vi "sv_Integrate and Differentiate Units.vi"(5 "integration type":T1(ring)=enum."none", 7 "custom unit label in":string, 8 "engineering units in":T2 items=["custom..."=0, "V"=1, "A"=21, "C"=30, "pC"=31, "s"=32, "-"=29, "Pa"=2, "N"=20, "g"=3, "m/s^2"=4, "m/s"=5, "m"=6, "mm/s"=12, "mm"=13, "micron/s"=14, "micron"=15, "in/s^2"=7, "in/s"=8, "in"=9, "mil/s"=10, "mil"=11, "rad/s^2"=16, "rad/s"=17, "rad"=18, "deg/s^2"=26, "deg/s"=27, "deg"=28, "RPM"=22, "cycle/s^2"=23, "Hz"=24, "cycle"=25, "strain"=19], 9 "input value":dbl=1.0) -> (1 "custom unit label out":string, 2 "engineering units out":T2 items=["custom..."=0, "V"=1, "A"=21, "C"=30, "pC"=31, "s"=32, "-"=29, "Pa"=2, "N"=20, "g"=3, "m/s^2"=4, "m/s"=5, "m"=6, "mm/s"=12, "mm"=13, "micron/s"=14, "micron"=15, "in/s^2"=7, "in/s"=8, "in"=9, "mil/s"=10, "mil"=11, "rad/s^2"=16, "rad/s"=17, "rad"=18, "deg/s^2"=26, "deg/s"=27, "deg"=28, "RPM"=22, "cycle/s^2"=23, "Hz"=24, "cycle"=25, "strain"=19], 3 "output value":dbl)   [LabVIEW 2017]
uses:
  <vilib>/addons/_NISVFA/_Shared subVIs/Controls/svc_Engineering Units Text Ring.ctl
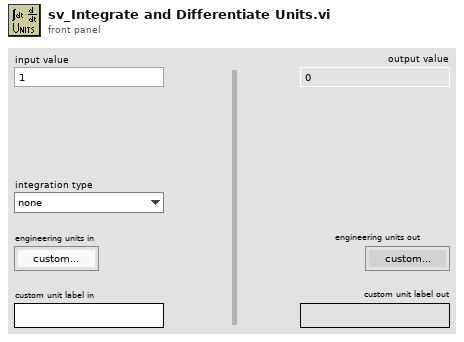
[diagram p1: front panel]
types:
  T1 = enum16{"single integration", "double integration", "single differentiation", "double differentiation", "none"}
  T2 = typedef "svc_Engineering Units Text Ring.ctl" = u16
  T3 = enum16{"custom...", "V", "Pa", "g", "m/s^2", "m/s", "m", "in/s^2", "in/s", "in", "mil/s", "mil", "mm/s", "mm", "micron/s", "micron", "rad/s^2", "rad/s", "rad", "strain", "N", "A", "rpm", "cycle/s^2", "Hz", "cycle", "deg/s^2", "deg/s", "deg", "Undefined", "C", "pC"}
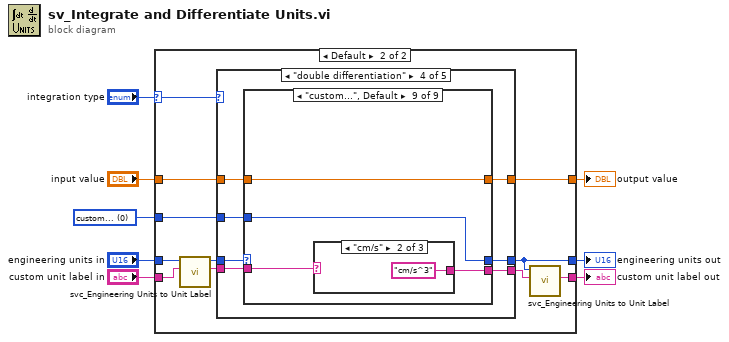
[diagram p0: block diagram]
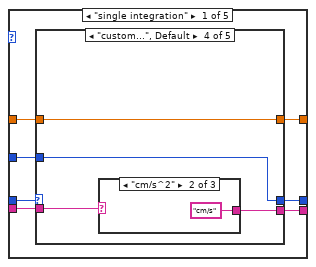
[diagram p3: hidden frame]
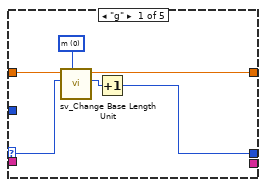
[diagram p4: hidden frame]
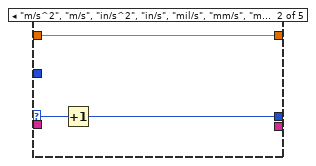
[diagram p5: hidden frame]
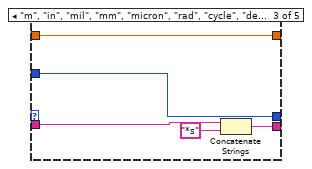
[diagram p6: hidden frame]
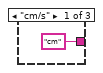
[diagram p7: hidden frame]
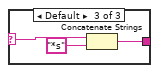
[diagram p8: hidden frame]
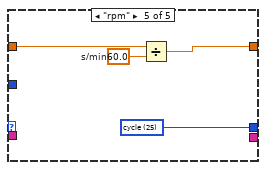
[diagram p9: hidden frame]
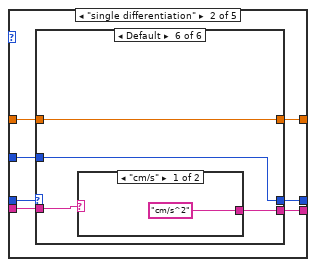
[diagram p10: hidden frame]
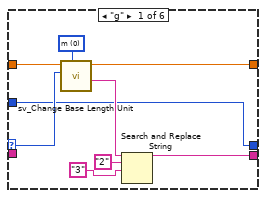
[diagram p11: hidden frame]
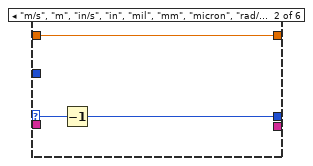
[diagram p12: hidden frame]
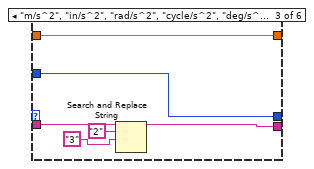
[diagram p13: hidden frame]
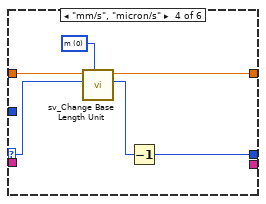
[diagram p14: hidden frame]
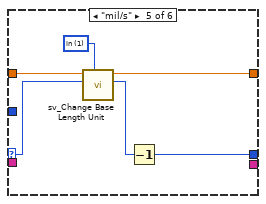
[diagram p15: hidden frame]
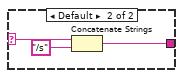
[diagram p16: hidden frame]
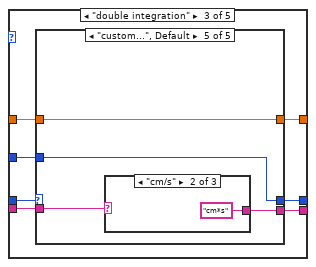
[diagram p17: hidden frame]
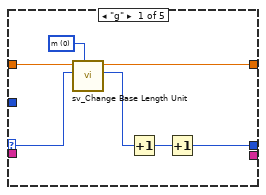
[diagram p18: hidden frame]
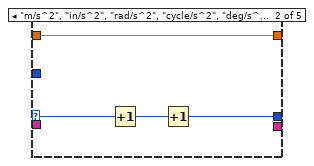
[diagram p19: hidden frame]
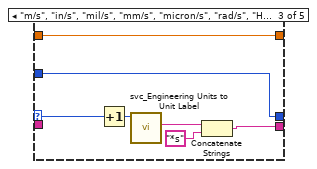
[diagram p20: hidden frame]
diagram:
  w1 = T2 0 items=["custom..."=0, "V"=1, "A"=21, "Pa"=2, "N"=20, "g"=3, "m/s^2"=4, "m/s"=5, "m"=6, "mm/s"=12, "mm"=13, "micron/s"=14, "micron"=15, "in/s^2"=7, "in/s"=8, "in"=9, "mil/s"=10, "mil"=11, "rad/s^2"=16, "rad/s"=17, "rad"=18, "deg/s^2"=26, "deg/s"=27, "deg"=28, "RPM"=22, "cycle/s^2"=23, "Hz"=24, "cycle"=25, "strain"=19] ("engineering units")
  n1 = case shown="Default" "integration type" {
    selector: "integration type" -> [_ w14]
    tunnel: [w9 w22] -> w8
    tunnel: [w10 w20] -> w7
    tunnel: "custom unit label in" -> [w9 w18]
    tunnel: [w11 w17] -> w5
    tunnel: "input value" -> [w11 w16]
    tunnel: "engineering units in" -> [w10 w13]
    tunnel: w1 -> [_ w12]
    frame "none" {
    }
    frame Default {
      n2 = call <vilib>:"svc_Engineering Units to Unit Label.vi"("custom label"=w18, "engineering units"=w13) -> ("unit label"=w19:string, "engineering units enum"=w15:T3)  [unwired: 8 in]
      n3 = case shown="\"double differentiation\"" w14 {
        tunnel: w15 -> [w29 w57 w108 w147 _]
        tunnel: [w28 w63 w107 w146 w221] -> w17
        tunnel: w16 -> [w27 w62 w106 w145 w221]
        tunnel: w19 -> [w26 w61 w105 w144 w220]
        tunnel: [w25 w60 w104 w143 _] -> w20
        tunnel: [w23 w58 w103 w142 w220] -> w21
        tunnel: w12 -> [w24 w59 w102 w141 _]
        frame "single integration" {
          n4 = case shown="\"custom...\", Default" w29 {
            selector: w29 -> [w32 w38 _ _ _]
            tunnel: [w34 w37 w39 w45 w53] -> w28
            tunnel: w27 -> [w35 w37 w39 w45 w54]
            tunnel: w26 -> [_ _ w40 w44 _]
            tunnel: [w33 w36 w42 w47 w56] -> w25
            tunnel: w24 -> [_ _ w42 w47 _]
            tunnel: [_ _ w41 w46 _] -> w23
            frame "g" {
              w31 = 0 items=["no change"=-1, "m"=0, "mm"=2, "microns"=3, "in"=1, "mils"=5] ("desired base units for length")
              n5 = call <vilib>:"sv_Change Base Length Unit.vi"("desired base units for vibration"=w31, "engineering units in"=w32, "value in [EU]"=w35) -> ("engineering units out"=w30:T2, "value out [desired EU]"=w34:dbl)  [unwired: 4 in, 1 out]
              n6 = Increment(x=w30) -> (x+1=w33:T2)
            }
            frame "m/s^2", "m/s", "in/s^2", "in/s", "mil/s", "mm/s", "micron/s", "rad/s^2", "rad/s", "cycle/s^2", "Hz", "deg/s^2", "deg/s" {
              n7 = Increment(x=w38) -> (x+1=w36:T3)
            }
            frame "m", "in", "mil", "mm", "micron", "rad", "cycle", "deg" {
              n8 = Concatenate Strings(w40, "*s" ("Input Element")) -> (w41:string)
            }
            frame "custom...", Default {
              n9 = case shown="\"cm/s^2\"" w44 {
                selector: w44 -> [_ _ w50]
                tunnel: ["cm" "cm/s" w51] -> w46
                frame "cm/s" {
                }
                frame "cm/s^2" {
                }
                frame Default {
                  n10 = Concatenate Strings(w50, "*s" ("Input Element")) -> (w51:string)
                }
              }
            }
            frame "rpm" {
              w55 = 60.0  # s/min
              w56 = T2 25 items=["custom..."=0, "V"=1, "A"=21, "Pa"=2, "N"=20, "g"=3, "m/s^2"=4, "m/s"=5, "m"=6, "mm/s"=12, "mm"=13, "micron/s"=14, "micron"=15, "in/s^2"=7, "in/s"=8, "in"=9, "mil/s"=10, "mil"=11, "rad/s^2"=16, "rad/s"=17, "rad"=18, "deg/s^2"=26, "deg/s"=27, "deg"=28, "RPM"=22, "cycle/s^2"=23, "Hz"=24, "cycle"=25, "strain"=19] ("engineering units")
              n11 = Divide(x=w54, y=w55) -> (x/y=w53:dbl)
            }
          }
        }
        frame "single differentiation" {
          n12 = case shown="Default" w57 {
            selector: w57 -> [w69 w75 _ w84 w90 _]
            tunnel: [w71 w74 w80 w86 w92 w95] -> w63
            tunnel: w62 -> [w72 w74 w80 w87 w93 w95]
            tunnel: w61 -> [_ _ w79 _ _ w94]
            tunnel: [w64 w73 w81 w82 w88 w97] -> w60
            tunnel: w59 -> [w64 _ w81 _ _ w97]
            tunnel: [w70 _ w78 _ _ w96] -> w58
            frame "g" {
              w68 = 0 items=["no change"=-1, "m"=0, "mm"=2, "microns"=3, "in"=1, "mils"=5] ("desired base units for length")
              n13 = call <vilib>:"sv_Change Base Length Unit.vi"("desired base units for vibration"=w68, "engineering units in"=w69, "value in [EU]"=w72) -> ("custom label out"=w65:string, "value out [desired EU]"=w71:dbl)  [unwired: 4 in, 1 out]
              n14 = Search and Replace String(input string=w65, search string="2", replace string="3" ("replace string (\"\")")) -> (result string=w70:string)  [unwired: 5 in, 3 out]
            }
            frame "m/s", "m", "in/s", "in", "mil", "mm", "micron", "rad/s", "rad", "Hz", "cycle", "deg/s", "deg" {
              n15 = Decrement(x=w75) -> (x-1=w73:T3)
            }
            frame "m/s^2", "in/s^2", "rad/s^2", "cycle/s^2", "deg/s^2" {
              n16 = Search and Replace String(input string=w79, search string="2", replace string="3" ("replace string (\"\")")) -> (result string=w78:string)  [unwired: 5 in, 3 out]
            }
            frame "mm/s", "micron/s" {
              w85 = 0 items=["no change"=-1, "g"=386, "m"=0, "cm"=4, "mm"=2, "microns"=3, "in"=1, "mils"=5] ("desired base units for vibration")
              n17 = call <vilib>:"sv_Change Base Length Unit.vi"("desired base units for vibration"=w85, "engineering units in"=w84, "value in [EU]"=w87) -> ("engineering units out"=w83:T2, "value out [desired EU]"=w86:dbl)  [unwired: 4 in, 1 out]
              n18 = Decrement(x=w83) -> (x-1=w82:T2)
            }
            frame "mil/s" {
              w91 = 1 items=["no change"=-1, "g"=386, "m"=0, "cm"=4, "mm"=2, "microns"=3, "in"=1, "mils"=5] ("desired base units for vibration")
              n19 = call <vilib>:"sv_Change Base Length Unit.vi"("desired base units for vibration"=w91, "engineering units in"=w90, "value in [EU]"=w93) -> ("engineering units out"=w89:T2, "value out [desired EU]"=w92:dbl)  [unwired: 4 in, 1 out]
              n20 = Decrement(x=w89) -> (x-1=w88:T2)
            }
            frame Default {
              n21 = case shown="\"cm/s\"" w94 {
                selector: w94 -> [_ w99]
                tunnel: ["cm/s^2" w100] -> w96
                frame "cm/s" {
                }
                frame Default {
                  n22 = Concatenate Strings(w99, "/s" ("Input Element")) -> (w100:string)
                }
              }
            }
          }
        }
        frame "double integration" {
          n23 = case shown="\"custom...\", Default" w108 {
            selector: w108 -> [w113 w118 w126 _ _]
            tunnel: [w115 w119 w125 w131 w135] -> w107
            tunnel: w106 -> [w114 w119 w125 w131 w135]
            tunnel: w105 -> [_ _ _ w127 w132]
            tunnel: [w109 w116 w124 w130 w134] -> w104
            tunnel: [_ _ w120 w129 w133] -> w103
            tunnel: w102 -> [_ _ w124 w130 w134]
            frame "g" {
              w112 = 0 items=["no change"=-1, "m"=0, "mm"=2, "microns"=3, "in"=1, "mils"=5] ("desired base units for length")
              n24 = call <vilib>:"sv_Change Base Length Unit.vi"("desired base units for vibration"=w112, "engineering units in"=w113, "value in [EU]"=w114) -> ("engineering units out"=w111:T2, "value out [desired EU]"=w115:dbl)  [unwired: 4 in, 1 out]
              n25 = Increment(x=w111) -> (x+1=w110:T2)
              n26 = Increment(x=w110) -> (x+1=w109:T2)
            }
            frame "m/s^2", "in/s^2", "rad/s^2", "cycle/s^2", "deg/s^2" {
              n27 = Increment(x=w118) -> (x+1=w117:T3)
              n28 = Increment(x=w117) -> (x+1=w116:T3)
            }
            frame "m/s", "in/s", "mil/s", "mm/s", "micron/s", "rad/s", "Hz", "deg/s" {
              n29 = Increment(x=w126) -> (x+1=w121:T3)
              n30 = call <vilib>:"svc_Engineering Units to Unit Label.vi"("engineering units"=w121) -> ("unit label"=w122:string)  [unwired: 9 in, 1 out]
              n31 = Concatenate Strings(w122, "*s" ("custom label")) -> (w120:string)
            }
            frame "m", "in", "mil", "mm", "micron", "rad", "cycle", "deg" {
              n32 = Concatenate Strings(w127, "*s^2" ("custom label")) -> (w129:string)
            }
            frame "custom...", Default {
              n33 = case shown="\"cm/s\"" w132 {
                selector: w132 -> [_ _ w138]
                tunnel: ["cm" "cm*s" w140] -> w133
                frame "cm/s^2" {
                }
                frame "cm/s" {
                }
                frame Default {
                  n34 = Concatenate Strings(w138, "*s^2" ("custom label")) -> (w140:string)
                }
              }
            }
          }
        }
        frame "double differentiation" {
          n35 = case shown="\"custom...\", Default" w147 {
            selector: w147 -> [w153 _ w170 w172 w183 w195 w199 w206 _]
            tunnel: [w156 w162 w169 w173 w184 w196 w200 w207 w212] -> w146
            tunnel: w145 -> [w155 w162 w169 w174 w185 w196 w201 w208 w212]
            tunnel: w144 -> [_ w158 _ _ _ _ _ _ w211]
            tunnel: [w154 w161 w168 w181 w192 w193 w202 w209 w213] -> w143
            tunnel: [w148 w157 w163 w176 w187 _ _ _ w214] -> w142
            tunnel: w141 -> [w154 w161 w168 w181 w192 _ _ _ w213]
            frame "g" {
              w152 = 0 items=["no change"=-1, "m"=0, "mm"=2, "microns"=3, "in"=1, "mils"=5] ("desired base units for length")
              n36 = call <vilib>:"sv_Change Base Length Unit.vi"("desired base units for vibration"=w152, "engineering units in"=w153, "value in [EU]"=w155) -> ("custom label out"=w149:string, "value out [desired EU]"=w156:dbl)  [unwired: 4 in, 1 out]
              n37 = Search and Replace String(input string=w149, search string="2", replace string="4" ("replace string (\"\")")) -> (result string=w148:string)  [unwired: 5 in, 3 out]
            }
            frame "m/s^2", "in/s^2", "rad/s^2", "cycle/s^2", "deg/s^2" {
              n38 = Search and Replace String(input string=w158, search string="2", replace string="4" ("replace string (\"\")")) -> (result string=w157:string)  [unwired: 5 in, 3 out]
            }
            frame "m/s", "in/s", "rad/s", "Hz", "deg/s" {
              n39 = Decrement(x=w170) -> (x-1=w167:T3)
              n40 = call <vilib>:"svc_Engineering Units to Unit Label.vi"("engineering units"=w167) -> ("unit label"=w164:string)  [unwired: 9 in, 1 out]
              n41 = Search and Replace String(input string=w164, search string="2", replace string="3" ("replace string (\"\")")) -> (result string=w163:string)  [unwired: 5 in, 3 out]
            }
            frame "mil/s" {
              w175 = 1 items=["no change"=-1, "g"=386, "m"=0, "cm"=4, "mm"=2, "micron"=3, "in"=1, "mil"=5] ("desired base units for vibration")
              n42 = call <vilib>:"sv_Change Base Length Unit.vi"("desired base units for vibration"=w175, "engineering units in"=w172, "value in [EU]"=w174) -> ("engineering units out"=w171:T2, "value out [desired EU]"=w173:dbl)  [unwired: 4 in, 1 out]
              n43 = Decrement(x=w171) -> (x-1=w180:T2)
              n44 = call <vilib>:"svc_Engineering Units to Unit Label.vi"("engineering units"=w180) -> ("unit label"=w177:string)  [unwired: 9 in, 1 out]
              n45 = Search and Replace String(input string=w177, search string="2", replace string="3" ("replace string (\"\")")) -> (result string=w176:string)  [unwired: 5 in, 3 out]
            }
            frame "mm/s", "micron/s" {
              w186 = 0 items=["no change"=-1, "g"=386, "m"=0, "cm"=4, "mm"=2, "micron"=3, "in"=1, "mil"=5] ("desired base units for vibration")
              n46 = call <vilib>:"sv_Change Base Length Unit.vi"("desired base units for vibration"=w186, "engineering units in"=w183, "value in [EU]"=w185) -> ("engineering units out"=w182:T2, "value out [desired EU]"=w184:dbl)  [unwired: 4 in, 1 out]
              n47 = Decrement(x=w182) -> (x-1=w191:T2)
              n48 = call <vilib>:"svc_Engineering Units to Unit Label.vi"("engineering units"=w191) -> ("unit label"=w188:string)  [unwired: 9 in, 1 out]
              n49 = Search and Replace String(input string=w188, search string="2", replace string="3" ("replace string (\"\")")) -> (result string=w187:string)  [unwired: 5 in, 3 out]
            }
            frame "m", "in", "rad", "cycle", "deg" {
              n50 = Decrement(x=w195) -> (x-1=w194:T3)
              n51 = Decrement(x=w194) -> (x-1=w193:T3)
            }
            frame "mil" {
              w198 = 1 items=["no change"=-1, "g"=386, "m"=0, "cm"=4, "mm"=2, "micron"=3, "in"=1, "mil"=5] ("desired base units for vibration")
              n52 = call <vilib>:"sv_Change Base Length Unit.vi"("desired base units for vibration"=w198, "engineering units in"=w199, "value in [EU]"=w201) -> ("engineering units out"=w197:T2, "value out [desired EU]"=w200:dbl)  [unwired: 4 in, 1 out]
              n53 = Decrement(x=w197) -> (x-1=w203:T2)
              n54 = Decrement(x=w203) -> (x-1=w202:T2)
            }
            frame "mm", "micron" {
              w205 = 0 items=["no change"=-1, "g"=386, "m"=0, "cm"=4, "mm"=2, "micron"=3, "in"=1, "mil"=5] ("desired base units for vibration")
              n55 = call <vilib>:"sv_Change Base Length Unit.vi"("desired base units for vibration"=w205, "engineering units in"=w206, "value in [EU]"=w208) -> ("engineering units out"=w204:T2, "value out [desired EU]"=w207:dbl)  [unwired: 4 in, 1 out]
              n56 = Decrement(x=w204) -> (x-1=w210:T2)
              n57 = Decrement(x=w210) -> (x-1=w209:T2)
            }
            frame "custom...", Default {
              n58 = case shown="\"cm/s\"" w211 {
                selector: w211 -> [_ _ w217]
                tunnel: ["cm/s^2" "cm/s^3" w218] -> w214
                frame "cm" {
                }
                frame "cm/s" {
                }
                frame Default {
                  n59 = Concatenate Strings(w217, "/s^2" ("Input Element")) -> (w218:string)
                }
              }
            }
          }
        }
        frame "none", Default {
        }
      }
      n60 = call <vilib>:"svc_Engineering Units to Unit Label.vi"("custom label"=w21, "engineering units"=w20) -> ("unit label"=w22:string)  [unwired: 8 in, 1 out]
    }
  }
  "custom unit label out" <- w8
  "engineering units out" <- w7
  "output value" <- w5
